vi "LINAKParseStatReg1.vi"(11 "StatusRegister1":u16) -> (0 "PositionValid":bool, 1 "TimeValid":bool, 2 "Ready":bool, 3 "StatusString":string, 4 "GoodToGo":bool)   [LabVIEW 2017]
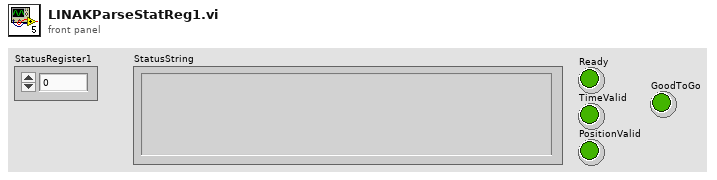
[diagram p1: front panel]
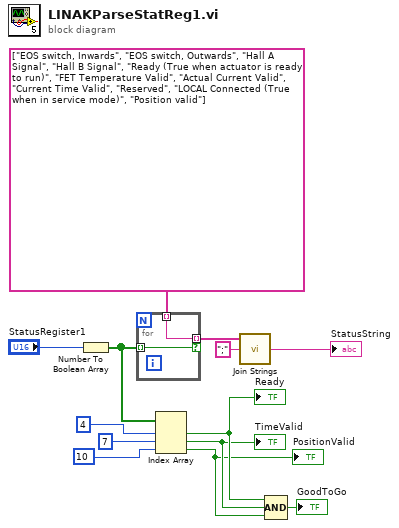
[diagram p0: block diagram]
diagram:
  n1 = Number To Boolean Array(number="StatusRegister1") -> (Boolean array=w8:bool[])
  n2 = for {
    tunnel: [w15] -> w11 mode=indexing if=w14
    tunnel: string[] ["EOS switch, Inwards", "EOS switch, Outwards", "Hall A Signal", "Hall B Signal", "Ready (True when actuator is ready to run)", "FET Temperature Valid", "Actual Current Valid", "Current Time Valid", "Reserved", "LOCAL Connected (True when in service mode)", "Position valid"] -> [w15] mode=indexing
    tunnel: w8 -> [w14] mode=indexing
  }
  n3 = Index Array(array=w8, index #1=4 ("index"), index #2=7 ("index"), index #3=10 ("index")) -> (element #1=w4:bool, element #2=w3:bool, element #3=w2:bool)
  "Ready" <- w4
  "TimeValid" <- w3
  "PositionValid" <- w2
  n4 = call <vilib>:"Join Strings.vi"("Separator (,)"=";", "Strings In"=w11) -> ("String"=→"StatusString":string)  [unwired: 1 in]
  n5 = Compound Arithmetic op=AND(w4, w3, w2) -> (→"GoodToGo":bool)
